vi "example_03_extract_specific.vi"() -> ()   [LabVIEW 2015, in "lv-bin-7zip.lvlib" / "v1.lvlib"]
uses:
  v1.lvlib
  <userlib>/antonio-alexander/lv-bin/lv-bin/public/api/v1/advanced/add_data_path_multiple.vi
  advanced/extract_exe_archive.vi
  advanced/extract_exe_specific.vi
  <userlib>/antonio-alexander/lv-bin/lv-bin/public/api/v1/v1.lvlib
panel:
  out "files_in_archive []":path[](array[path])
  in  "files_to_extract (relative) []":path[](array[path])
  out "target_path out":path
  out "archive_path out":path
  out "files []":path[](array[path])
  out "error out":errorcluster
  in  "target_path in":path
  in  "archive_path":path
  in  "bin_path":path
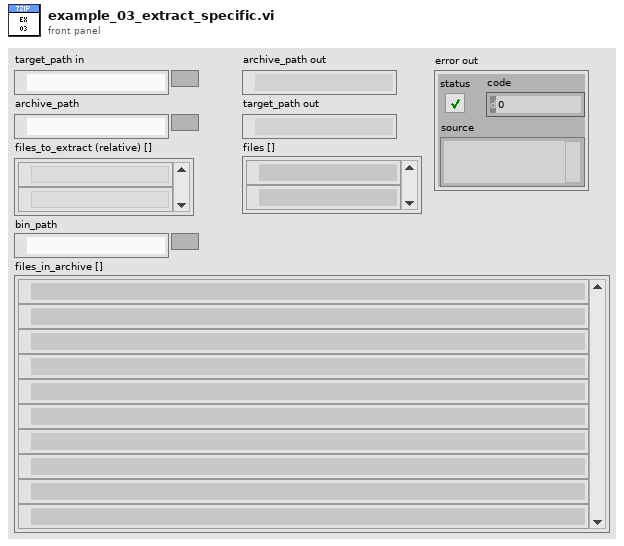
[diagram p1: front panel]
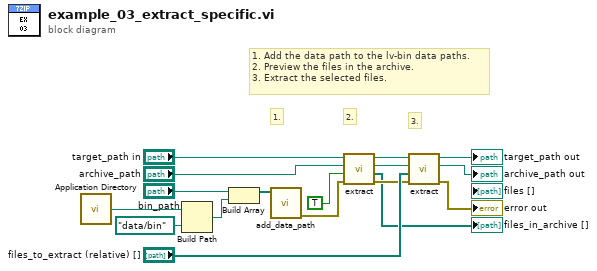
[diagram p0: block diagram]
diagram:
  # "3."
  # "1."
  # "1. Add the data path to the lv-bin data paths.\n2. Preview the files in the archive.\n3. Extract the selected files."
  # "2."
  n1 = call <vilib>:"Application Directory.vi"() -> ("Application Directory"=w14:path)
  n2 = Build Path(base path=w14, name or relative path=path "data/bin" ("Application Directory")) -> (appended path=w15:path)
  n3 = Build Array("bin_path", w15) -> (w16:path[])
  n4 = call-poly <userlib>:"add_data_path.vi"("path_to_add []"=w16) -> ("error out"=w3:errorcluster)  [unwired: 10 in]
  n5 = call-poly "extract.vi"("error in (no error)"=w3, "preview?"=TRUE, "archive_path"="archive_path", "target_path in"="target_path in") -> ("error out"=w2:errorcluster, "files []"=→"files_in_archive []":path[], "archive_path out"=w7:path, "target_path out"=w5:path)  [unwired: 4 in]
  n6 = call-poly "extract.vi"("error in (no error)"=w2, "files_to_extract (relative) []"="files_to_extract (relative) []", "target_path in"=w7, "archive_path (file_dialog)"=w5) -> ("error out"=→"error out":errorcluster, "target_path out"=→"archive_path out":path, "archive_path out"=→"target_path out":path)  [unwired: 5 in]
